vi "gyro -- async fitter.vi"(11 "server event pair":T9) -> ()   [LabVIEW 2018]
uses:
  plot refs -- filter related.ctl
  cursor window action.ctl
  publisher action.ctl
  cursor action.ctl
  2Dwindow.ctl
  server talkback message type.ctl
  circle corners.ctl
  lorentzian.ctl
  peak -- parameters -- complex fit.ctl
  wavepacket.ctl
  filter method control.ctl
  show-win- control.ctl
  server talkto message type.ctl
  server talk-to-back pair.ctl
panel:
  in  "Tab :  Fit controls":T1(tab)
  out "lorentzian":T2={"A (VHz)"=0.005614170164837037, "f (Hz)"=70488.63611178169, "G (Hz)"=428.0110281609372, "phi(rad)"=4.459926465221261, "Q"=164.68883153467982, "Norm  Ampl"=nan, "bg (V)"=2.8688017502385223e-05+0.00035144607353619194i, "4corners"={"z (-pi/2)"=1.2710482317097233e-05+0.00034202144845651717i, "z(inf)"=2.8688017502385223e-05+0.00035144607353619194i, "z (pi/2)"=1.9263392422710455e-05+0.00036742360872147993i, "z center"=1.5986937369903844e-05+0.00035472252858899855i, "z(0)"=3.2858572374224653e-06+0.00035799898364180516i, "radius"=1.3116882032128489e-05}} {"bg (V)" format="%#9_9f"; "Q" format="%#9_9f"; "phi(rad)" format="%#9_9f"; "G (Hz)" format="%#9_9f"; "f (Hz)" format="%#9_9f"}
  in  "Plot: fragment - filter":cluster{dbl[], dbl[]}[](graph)=[{array[298 elements], array[298 elements]}, {array[298 elements], array[298 elements]}, {array[298 elements], array[298 elements]}, {array[298 elements], array[298 elements]}]
  out "Plot: phase around center":cluster{dbl[], dbl[]}[](graph)
  out "Plot: fragment":cluster{dbl[], dbl[]}[](graph)
  out "Plot: complex plane":cluster{dbl[], dbl[]}[](graph)=[{array[298 elements], array[298 elements]}, {[2.9103819402032333e-05, 2.900038886938624e-05, 2.8691728432734196e-05, 2.8182705851547014e-05, 2.748134871600537e-05, 2.6598717847107188e-05, 2.5548732860913123e-05, 2.4347952647886086e-05, 2.301531422929684e-05, 2.1571834109086143e-05, 2.0040276831042943e-05, 1.844479596834995e-05, 1.6810553207305906e-05, 1.516332153250178e-05, 1.3529078771457734e-05, 1.1933597908764745e-05, 1.0402040630721545e-05, 8.958560510510845e-06, 7.625922091921602e-06, 6.4251418788945635e-06, 5.375156892700502e-06, 4.492526023802321e-06, 3.791168888260671e-06, 3.28214630707349e-06, 2.9734858704214465e-06, 2.8700553377753553e-06, 2.973485870421448e-06, 3.28214630707349e-06, 3.7911688882606744e-06, 4.492526023802321e-06, 5.3751568927005036e-06, 6.425141878894565e-06, 7.625922091921604e-06, 8.958560510510852e-06, 1.0402040630721552e-05, 1.1933597908764745e-05, 1.3529078771457736e-05, 1.5163321532501782e-05, 1.6810553207305913e-05, 1.844479596834996e-05, 2.004027683104294e-05, 2.1571834109086143e-05, 2.301531422929684e-05, 2.434795264788609e-05, 2.554873286091313e-05, 2.659871784710719e-05, 2.748134871600537e-05, 2.8182705851547017e-05, 2.86917284327342e-05, 2.9000388869386243e-05], [0.00035472252858899855, 0.00035636650982836675, 0.0003579845645015233, 0.00035955117491969353, 0.0003610416347007352, 0.0003624324384035438, 0.0003637016522229001, 0.00036482925989868135, 0.00036579747838424027, 0.00036659103829567386, 0.00036719742471912916, 0.00036760707457847056, 0.0003678135274507033, 0.0003678135274507033, 0.00036760707457847056, 0.00036719742471912916, 0.00036659103829567386, 0.00036579747838424027, 0.00036482925989868135, 0.0003637016522229001, 0.0003624324384035438, 0.0003610416347007352, 0.00035955117491969353, 0.0003579845645015233, 0.00035636650982836675, 0.00035472252858899855, 0.00035307854734963035, 0.0003514604926764738, 0.00034989388225830357, 0.0003484034224772619, 0.0003470126187744533, 0.000345743404955097, 0.00034461579727931575, 0.00034364757879375683, 0.00034285401888232324, 0.00034224763245886794, 0.00034183798259952654, 0.0003416315297272938, 0.0003416315297272938, 0.00034183798259952654, 0.00034224763245886794, 0.00034285401888232324, 0.00034364757879375683, 0.00034461579727931575, 0.000345743404955097, 0.0003470126187744533, 0.0003484034224772619, 0.00034989388225830357, 0.0003514604926764738, 0.00035307854734963035]}, {[2.8688017502385223e-05, 2.7417909489137084e-05, 2.6147801475888948e-05, 2.487769346264081e-05, 2.3607585449392673e-05, 2.2337477436144533e-05, 2.1067369422896394e-05, 1.9797261409648255e-05, 1.852715339640012e-05, 1.7257045383151983e-05, 1.5986937369903844e-05, 1.4716829356655705e-05, 1.3446721343407567e-05, 1.217661333015943e-05, 1.090650531691129e-05, 9.636397303663155e-06, 8.366289290415015e-06, 7.096181277166876e-06, 5.82607326391874e-06, 4.555965250670601e-06], [0.00035144607353619194, 0.0003517737190414726, 0.00035210136454675325, 0.00035242901005203394, 0.00035275665555731456, 0.00035308430106259525, 0.00035341194656787593, 0.00035373959207315656, 0.00035406723757843724, 0.00035439488308371787, 0.00035472252858899855, 0.00035505017409427923, 0.00035537781959955986, 0.00035570546510484054, 0.00035603311061012117, 0.00035636075611540185, 0.00035668840162068254, 0.00035701604712596316, 0.00035734369263124385, 0.0003576713381365245]}, {[1.2710482317097233e-05, 1.3038127822377894e-05, 1.3365773327658556e-05, 1.3693418832939216e-05, 1.4021064338219878e-05, 1.4348709843500539e-05, 1.4676355348781199e-05, 1.5004000854061861e-05, 1.5331646359342523e-05, 1.5659291864623182e-05, 1.5986937369903844e-05, 1.6314582875184506e-05, 1.6642228380465168e-05, 1.6969873885745827e-05, 1.729751939102649e-05, 1.7625164896307148e-05, 1.795281040158781e-05, 1.8280455906868472e-05, 1.8608101412149134e-05, 1.8935746917429793e-05], [0.00034202144845651717, 0.0003432915564697653, 0.00034456166448301344, 0.00034583177249626157, 0.0003471018805095097, 0.0003483719885227579, 0.000349642096536006, 0.00035091220454925415, 0.0003521823125625023, 0.0003534524205757504, 0.00035472252858899855, 0.0003559926366022467, 0.0003572627446154948, 0.00035853285262874295, 0.0003598029606419911, 0.0003610730686552392, 0.0003623431766684874, 0.00036361328468173553, 0.00036488339269498366, 0.0003661535007082318]}, {[-0.12051735461029346, -0.12207348598889368, -0.12355331127335088, -0.1249559056210327, -0.1262803924561282, -0.1275259440174794, -0.12869178187590485, -0.12977717742069275, -0.13078145231495877, -0.1317039789195845, -0.1325441806854716, -0.13330153251386614, -0.13397556108452827, -0.13456584515154188, -0.13507201580657965, -0.13549375670945876, -0.13583080428584318, -0.13608294789196904, -0.13625002994629012, -0.13633194602796123], [0.06411190542991022, 0.061078796354348035, 0.05800773584383981, 0.05490064321123721, 0.0517594602882955, 0.04858615021209154, 0.045382696198127265, 0.04215110030088447, 0.03889338216260588, 0.03561157775108473, 0.03230773808725083, 0.02898392796334944, 0.02564222465251332, 0.022284716610534536, 0.018913502170647845, 0.015530688232140346, 0.012138388943608257, 0.008738724381682807, 0.005333819226051277, 0.0019258014316016106]}, {[-0.13377675222220706, -0.1355040580524533, -0.1371466641182008, -0.1387035438441276, -0.14017372423108362, -0.14155628646418342, -0.1428503664870357, -0.14405515554175027, -0.14516990067438554, -0.14619390520552009, -0.14712652916565477, -0.14796718969517272, -0.14871536140860767, -0.14937057672299278, -0.1499324261500847, -0.15040055855228054, -0.15077468136206723, -0.15105456076486692, -0.15124002184516333, -0.15133094869581826], [0.07112534787775143, 0.0677585968038774, 0.06434971963721327, 0.06090084681502438, 0.05741413377055908, 0.05389175958597269, 0.050335925630472345, 0.04674885418453284, 0.0431327870510436, 0.03948998415425513, 0.0358227221273995, 0.032133292889868964, 0.02842400221484086, 0.024697168288244413, 0.020955120259970185, 0.01720019678822686, 0.013434744577956244, 0.009661116914218993, 0.005881672191467993, 0.0020987724396288633]}, {array[298 elements], array[298 elements]}]
  in  "scale gauge: Plot: complex plane":dbl(slide)=0.00275 min=0.0 max=0.3 step=1e-06 scale=1e-05..0.5 scale format="%#_3p"
  out "Plot: phase":cluster{"omega out":dbl[], dbl[]}(graph)
  out "Plot: win omega":T4(graph)
  out "Plot: dz/domega":cluster{"omega out":dbl[], dbl[]}(graph)
  in  "Plot: complex plane - filter":cluster{dbl[], dbl[]}[](graph)=[{array[298 elements], array[298 elements]}, {array[298 elements], array[298 elements]}, {[2.905030396515612e-05, 2.9022632451479088e-05, 2.893972711727057e-05, 2.8801915152008838e-05, 2.8609740436560477e-05, 2.8363961396731098e-05, 2.8065548010105136e-05, 2.77156779779875e-05, 2.731573207755454e-05, 2.6867288712557366e-05, 2.6372117684083335e-05, 2.5832173205959713e-05, 2.5249586192364487e-05, 2.4626655848081624e-05, 2.3965840594590203e-05, 2.326974836779799e-05, 2.2541126325709838e-05, 2.1782850006650124e-05, 2.099791198082668e-05, 2.018941004002336e-05, 1.9360534972031112e-05, 1.8514557968066298e-05, 1.7654817712873437e-05, 1.6784707208461826e-05, 1.5907660383476688e-05, 1.5027138541051666e-05, 1.4146616698626644e-05, 1.3269569873641507e-05, 1.2399459369229891e-05, 1.1539719114037038e-05, 1.0693742110072223e-05, 9.864867042079974e-06, 9.056365101276651e-06, 8.271427075453208e-06, 7.513150756393494e-06, 6.784528714305347e-06, 6.088436487513131e-06, 5.427621234021711e-06, 4.804690889738847e-06, 4.222103876143618e-06, 3.682159398019999e-06, 3.1869883695459693e-06, 2.7385450045487964e-06, 2.338599104115837e-06, 1.988729071998198e-06, 1.690315685372236e-06, 1.4445366455428568e-06, 1.252361930094499e-06, 1.1145499648327652e-06, 1.0316446306242462e-06, 1.0039731169472153e-06, 1.0316446306242462e-06, 1.1145499648327669e-06, 1.252361930094499e-06, 1.4445366455428568e-06, 1.6903156853722394e-06, 1.9887290719982014e-06, 2.338599104115837e-06, 2.738545004548798e-06, 3.186988369545971e-06, 3.6821593980200005e-06, 4.2221038761436245e-06, 4.8046908897388484e-06, 5.427621234021715e-06, 6.088436487513134e-06, 6.784528714305345e-06, 7.513150756393502e-06, 8.27142707545321e-06, 9.05636510127666e-06, 9.864867042079978e-06, 1.0693742110072223e-05, 1.1539719114037043e-05, 1.2399459369229895e-05, 1.3269569873641516e-05, 1.4146616698626647e-05, 1.5027138541051664e-05, 1.5907660383476695e-05, 1.6784707208461826e-05, 1.7654817712873447e-05, 1.8514557968066298e-05, 1.936053497203111e-05, 2.0189410040023365e-05, 2.099791198082668e-05, 2.178285000665013e-05, 2.254112632570984e-05, 2.3269748367798e-05, 2.396584059459021e-05, 2.4626655848081624e-05, 2.5249586192364494e-05, 2.5832173205959716e-05, 2.6372117684083342e-05, 2.6867288712557366e-05, 2.731573207755454e-05, 2.77156779779875e-05, 2.806554801010514e-05, 2.83639613967311e-05, 2.860974043656048e-05, 2.8801915152008838e-05, 2.893972711727057e-05, 2.9022632451479088e-05], [0.0003546065647290071, 0.00035548708657143213, 0.00035636413339641725, 0.00035723424390082884, 0.00035809398415602173, 0.0003589399611599865, 0.0003597688362279788, 0.0003605773381687821, 0.00036136227619460554, 0.00036212055251366525, 0.0003628491745557534, 0.0003635452667825456, 0.00036420608203603704, 0.0003648290123803199, 0.00036541159939391515, 0.00036595154387203876, 0.0003664467149005128, 0.00036689515826550997, 0.0003672951041659429, 0.0003676449741980606, 0.00036794338758468654, 0.0003681891666245159, 0.00036838134133996425, 0.000368519153305226, 0.0003686020586394345, 0.00036862973015311157, 0.0003686020586394345, 0.000368519153305226, 0.00036838134133996425, 0.0003681891666245159, 0.00036794338758468654, 0.0003676449741980606, 0.0003672951041659429, 0.00036689515826550997, 0.0003664467149005128, 0.00036595154387203876, 0.00036541159939391515, 0.0003648290123803199, 0.00036420608203603704, 0.0003635452667825456, 0.0003628491745557534, 0.00036212055251366525, 0.00036136227619460554, 0.0003605773381687821, 0.0003597688362279788, 0.0003589399611599865, 0.00035809398415602173, 0.00035723424390082884, 0.00035636413339641725, 0.00035548708657143213, 0.0003546065647290071, 0.00035372604288658204, 0.0003528489960615969, 0.00035197888555718533, 0.00035111914530199244, 0.00035027316829802765, 0.0003494442932300354, 0.0003486357912892321, 0.00034785085326340863, 0.0003470925769443489, 0.00034636395490226076, 0.00034566786267546857, 0.00034500704742197714, 0.00034438411707769426, 0.00034380153006409903, 0.0003432615855859754, 0.0003427664145575014, 0.0003423179711925042, 0.00034191802529207125, 0.0003415681552599536, 0.00034126974187332764, 0.0003410239628334983, 0.0003408317881180499, 0.0003406939761527882, 0.0003406110708185797, 0.0003405833993049026, 0.0003406110708185797, 0.0003406939761527882, 0.0003408317881180499, 0.0003410239628334983, 0.00034126974187332764, 0.0003415681552599536, 0.00034191802529207125, 0.0003423179711925042, 0.0003427664145575014, 0.0003432615855859754, 0.00034380153006409903, 0.00034438411707769426, 0.00034500704742197714, 0.00034566786267546857, 0.00034636395490226076, 0.0003470925769443489, 0.00034785085326340863, 0.0003486357912892321, 0.0003494442932300354, 0.00035027316829802765, 0.00035111914530199244, 0.00035197888555718533, 0.0003528489960615969, 0.00035372604288658204]}, {[3.4550485346656053e-06, -7.59654128881755e-06, 4.382620039101754e-06], [-5.3982458510331535e-06, 1.2688424660565133e-06, -1.3270376410500222e-06]}, {[3.6013253466750408e-06, 3.652728139630199e-06, 3.704130932585357e-06, 3.7555337255405156e-06, 3.806936518495674e-06, 3.858339311450832e-06, 3.909742104405991e-06, 3.961144897361148e-06, 4.012547690316307e-06, 4.063950483271465e-06, 4.115353276226624e-06, 4.166756069181782e-06, 4.21815886213694e-06, 4.269561655092099e-06, 4.320964448047256e-06, 4.372367241002415e-06, 4.423770033957573e-06, 4.475172826912732e-06, 4.52657561986789e-06, 4.5779784128230484e-06], [-4.818979876248634e-06, -4.62743245445747e-06, -4.435885032666307e-06, -4.244337610875143e-06, -4.0527901890839785e-06, -3.861242767292814e-06, -3.669695345501651e-06, -3.478147923710487e-06, -3.2866005019193234e-06, -3.0950530801281598e-06, -2.9035056583369957e-06, -2.711958236545832e-06, -2.5204108147546683e-06, -2.3288633929635042e-06, -2.1373159711723406e-06, -1.9457685493811765e-06, -1.7542211275900128e-06, -1.5626737057988492e-06, -1.371126284007685e-06, -1.1795788622165214e-06]}, {[-7.59654128881755e-06, -7.4016964168323305e-06, -7.206851544847112e-06, -7.012006672861892e-06, -6.817161800876673e-06, -6.6223169288914536e-06, -6.427472056906234e-06, -6.232627184921015e-06, -6.0377823129357955e-06, -5.842937440950577e-06, -5.648092568965357e-06, -5.453247696980138e-06, -5.2584028249949185e-06, -5.063557953009699e-06, -4.86871308102448e-06, -4.6738682090392604e-06, -4.479023337054041e-06, -4.284178465068822e-06, -4.089333593083603e-06, -3.894488721098383e-06], [1.2688424660565133e-06, 1.2688424660565133e-06, 1.2688424660565133e-06, 1.2688424660565133e-06, 1.2688424660565133e-06, 1.2688424660565133e-06, 1.2688424660565133e-06, 1.2688424660565133e-06, 1.2688424660565133e-06, 1.2688424660565133e-06, 1.2688424660565133e-06, 1.2688424660565133e-06, 1.2688424660565133e-06, 1.2688424660565133e-06, 1.2688424660565133e-06, 1.2688424660565133e-06, 1.2688424660565133e-06, 1.2688424660565133e-06, 1.2688424660565133e-06, 1.2688424660565133e-06]}]
  in  "parameters -- scan monitor control.ctlparameters: complex fit":T5={"main VI path"=path "", "scale factor"=3.0, "# of grid points"=200, "parameters: wavepacket"={"R"=0.5, "wave number"=22.0, "delta k"=7.0, "radii vector"=[], "radial section"=[], "wave vector"=22.0, "wavepacket is"=TRUE}, "span"=0.27789, "interference ?"=enum."cp z center", "filter method"=enum."three"} {"span" min=0.0 max=0.5 step=1e-05 scale=0.0001..0.5 scale format="%#_5f"; "parameters: wavepacket"."delta k" format="%#_3f"; "parameters: wavepacket"."wave number" format="%#_3f"; "parameters: wavepacket"."R" format="%#_3f"}
  in  "win":T8={"cen (Hz)"=45005.0594236074, "win (Hz)"=127.23590686512762, "left (Hz)"=44941.44147017484, "right (Hz)"=45068.67737703997}
  out "circle frequency (Hz)":dbl=70488.63611178169 format="%#11_11f"
  out "circle gamma (Hz)":dbl=428.0110281609372 format="%#11_11f"
  out "circle phase (rad)":dbl=4.459926465221261 format="%#11_11f"
  out "circle Q":dbl=164.68883153467982 format="%#11_11f"
  in  "tab":enum32{"complex plane"}(tab)
  in  "plot staff!":enum16{"plot", "do not plot", "a"}(ring)
  in  "use fast fit!":bool
  out "# of points":dbl=953.475933538175
  out "win center (kHz)":dbl=3399.029286744401
  out "win width (kHz)":dbl=76.27809365793496
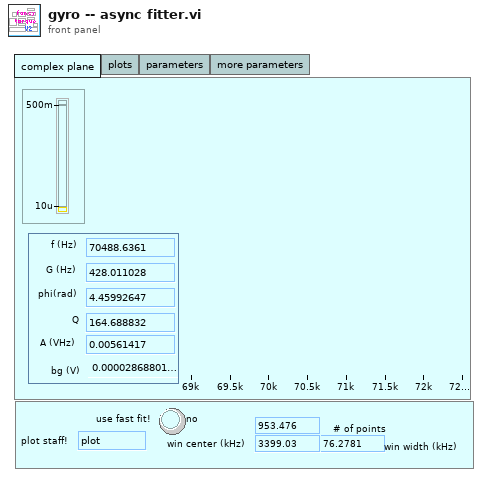
[diagram p1: front panel]
types:
  T1 = enum32{"complex plane", "plots", "parameters", "more parameters"}
  T2 = typedef "lorentzian.ctl" = cluster{"A (VHz)":dbl, "f (Hz)":dbl, "G (Hz)":dbl, "phi(rad)":dbl, "Q":dbl, "Norm  Ampl":dbl, "bg (V)":cdb, "4corners":T3}
  T3 = typedef "circle corners.ctl" = cluster{"z (-pi/2)":cdb, "z(inf)":cdb, "z (pi/2)":cdb, "z center":cdb, "z(0)":cdb, "radius":dbl}
  T4 = cluster{"omega out":dbl[], "win omega out":dbl[]}
  T5 = typedef "peak -- parameters -- complex fit.ctl" = cluster{"main VI path":path, "scale factor":dbl, "# of grid points":i32, "parameters: wavepacket":T6, "span":dbl, "interference ?":enum16{"cp z center", "pm zcenter", "fancy"}, "filter method":T7}
  T6 = typedef "wavepacket.ctl" = cluster{"R":dbl, "wave number":dbl, "delta k":dbl, "radii vector":dbl[], "radial section":cdb[], "wave vector":dbl, "wavepacket is":bool}
  T7 = typedef "filter method control.ctl" = enum16{"four", "five", "one", "two", "three", "zero", "minus one", "minus two"}
  T8 = typedef "show-win- control.ctl" = cluster{"cen (Hz)":dbl, "win (Hz)":dbl, "left (Hz)":dbl, "right (Hz)":dbl}
  T9 = typedef "server talk-to-back pair.ctl" = cluster{"talkback event":refnum<user-event>, "talkto event":refnum<user-event>}
  T10 = typedef "plot refs -- filter related.ctl" = cluster{"Plot: complex plane - filter":refnum<vi>, "Plot: dz/domega":refnum<vi>, "Plot: fragment filter":refnum<vi>, "Plot: win omega":refnum<vi>, "Plot: phase":refnum<vi>, "Plot: phase around center":refnum<vi>, "Plot: complex plane":refnum<vi>, "Plot: fragment":refnum<vi>}
  T11 = typedef "2Dwindow.ctl" = cluster{"window y":dbl, "center x":dbl, "center y":dbl, "window x":dbl}
  T12 = typedef "cursor action.ctl" = enum16{"range", "read", "write", "check", "zoom out", "smart zoom out", "zoom to aspect ratio 1", "zoom to win", "zoom out 20%", "zoom in 20%", "-empty", "smart zoom out&aspect", "move range left 20%", "move range right 20%", "move range up 20%", "move range down 20%", "zoom to X win", "zoom to Y win", "zoom out X", "zoom out Y", "zoom in X", "zoom in Y", "check plot scale"}
  T13 = typedef "cursor window action.ctl" = enum16{"balance", "h. offset change", "cursor moves", "change center", "change window", "init", "check", "reset", "set y to middle", "idle", "-write all Y", "-write left.X", "-write center.X", "-write right.X", "-write all X", "-change center", "-change window", "-change skew", "-read cursor 2", "-read cursor 1", "-read cursor 0", "-read all cursors", "-reset", "-read plot scale", "-set y to middle", "-Q: center.Y is visible", "-Q: window is visible", "-parse center.Y", "-right left from center", "-left move", "-right move", "-set center.Y", "-empty", "-set cursors to default", "-check", "-write center.Y", "-copy cursor 1", "-copy cursor 0", "-copy cursor 2", "move right", "move left", "shrink", "broaden", "skew up", "skew down", "-write plot scale", "zoom X", "change cen&win", "zoom to all data", "color--red", "color--green", "color--yellow", "read", "zoom out", "zoom in", "slide right", "slide left", "set range aspect ratio to 1"}
  T14 = typedef "eventvkey.ctl" = enum16{"ASCII", "Enter", "Return", "Shift", "Ctrl", "Alt", "Cmd", "Opt", "Caps", "NumLock", "Clear", "Break", "Up", "Down", "Left", "Right", "Insert", "Delete", "Home", "End", "PageUp", "PageDown", "Escape", "Help", "Pause", "ScrollLock", "F1", "F2", "F3", "F4", "F5", "F6", "F7", "F8", "F9", "F10", "F11", "F12", "F13", "F14", "F15", "F16", "F17", "F18", "F19", "F20", "F21", "F22", "F23", "F24", "Play", "VolumeUp", "VolumeDown", "Mute", "Two Byte Char"}
  T15 = typedef "publisher action.ctl" = enum16{"set", "get", "init", "check"}
  T16 = typedef "server talkback message type.ctl" = cluster{"message":enum16{"new", "void"}}
  T17 = typedef "cursor winow.ctl" = cluster{"left":dbl, "right ":dbl, "center":dbl, "window":dbl, "cursors":i32[], "relative":i32, "absolute":i32, "fixed vertical offset":dbl, "vertical offset":dbl, "skew":dbl, "default window frac":dbl, "kind":enum16{"symmetric", "skewed", "fancy"}, "skew.left":dbl, "skew.right":dbl, "Plot ref":refnum<vi>, "wing order":enum16{"forw", "back"}}
  T18 = enum16{"stop", "start", "update pars", "update request", "new", "launch", "exit", "get", "reset", "pause", "unpause"}
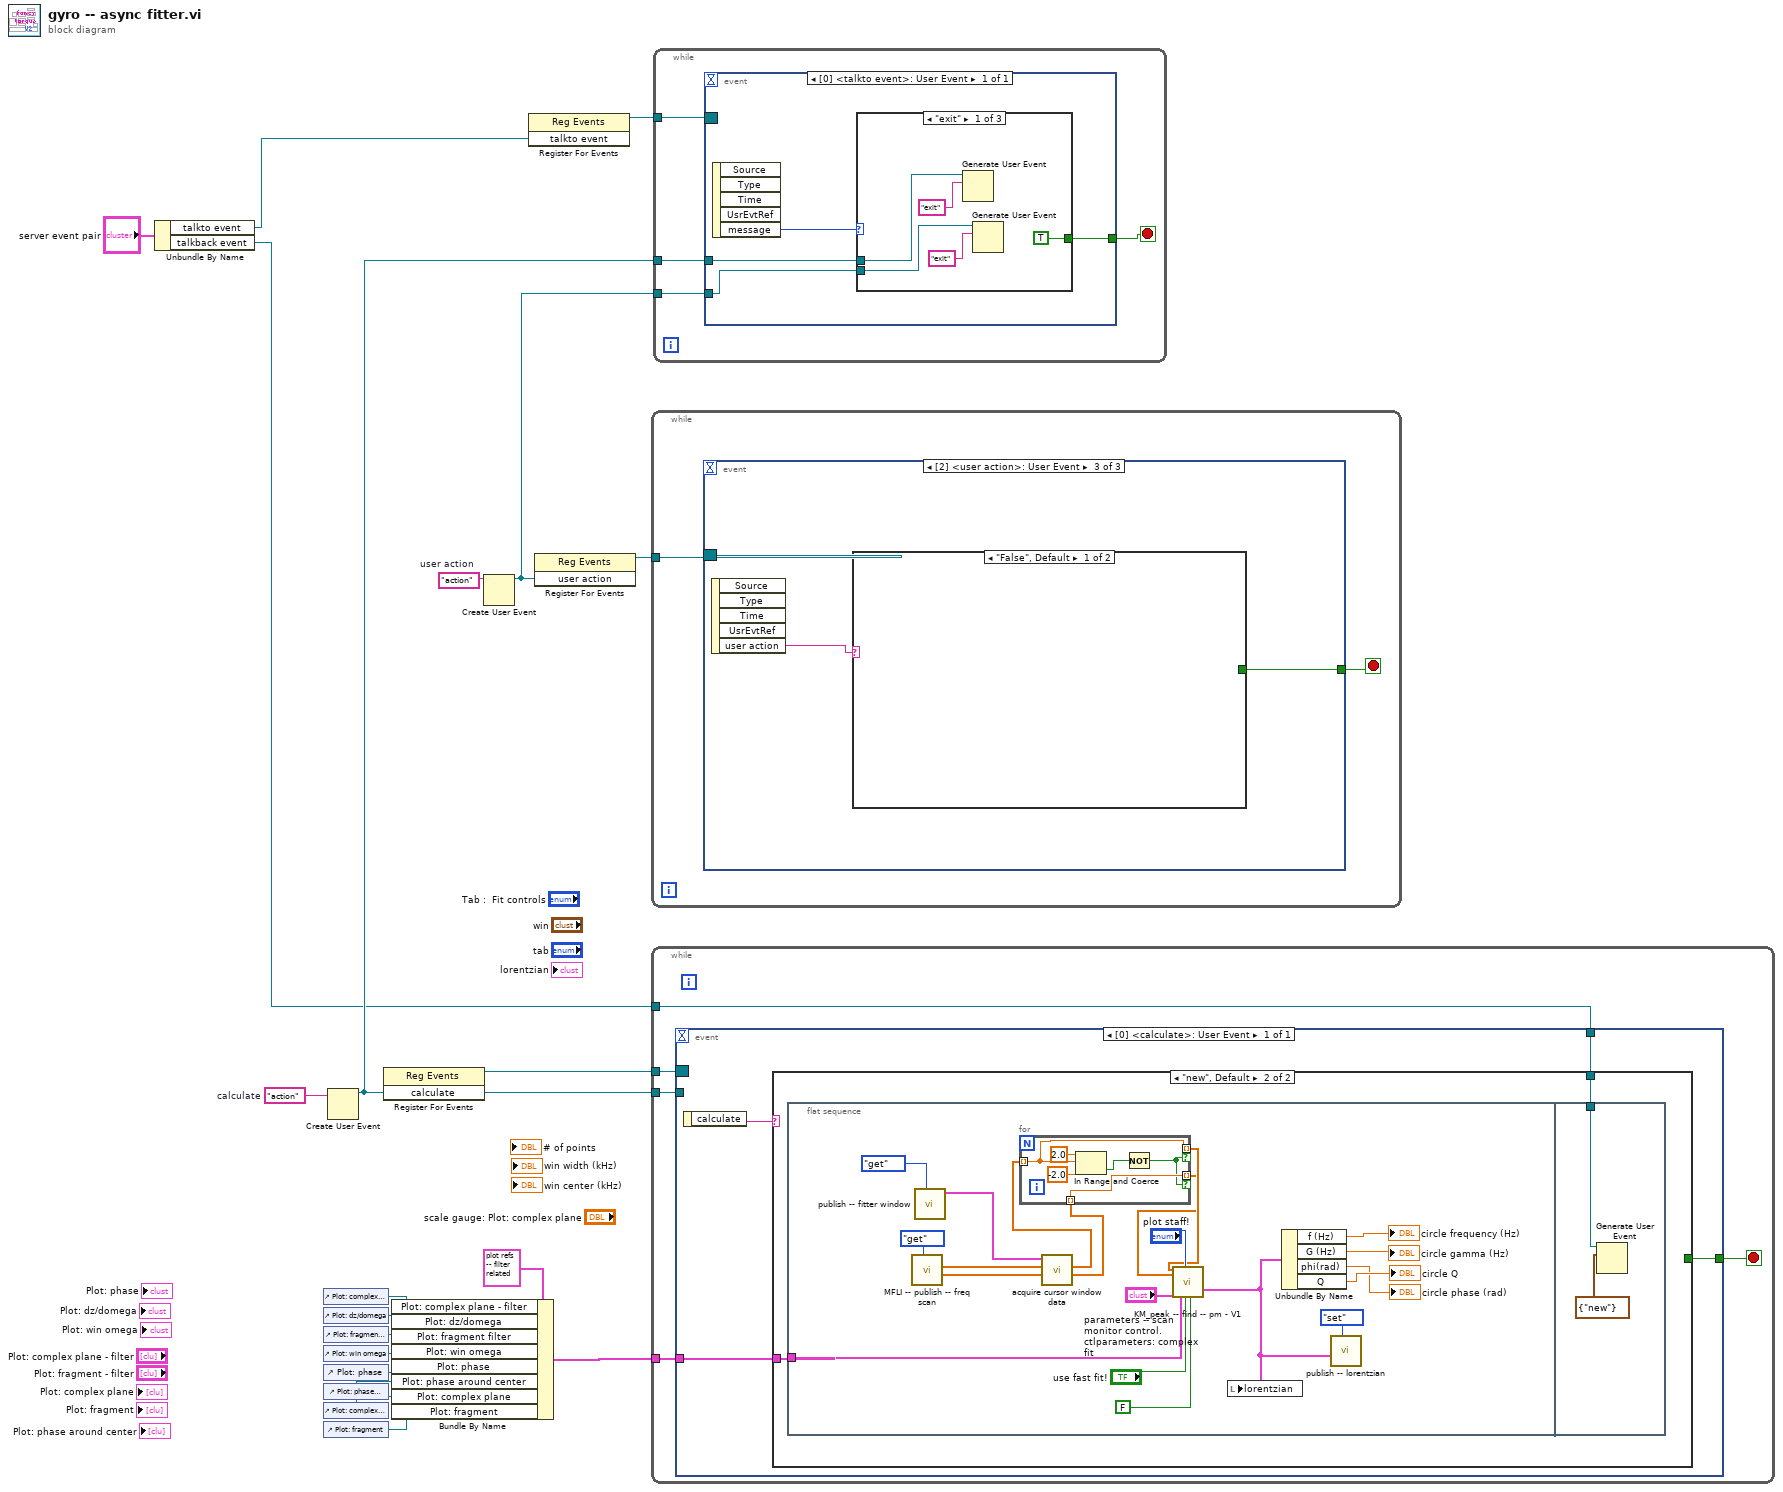
[diagram p0: block diagram]
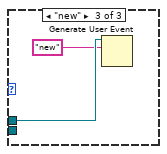
[diagram p3: hidden frame]
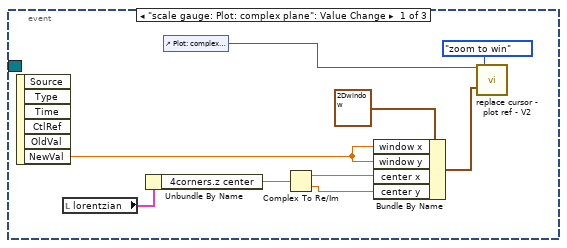
[diagram p4: hidden frame]
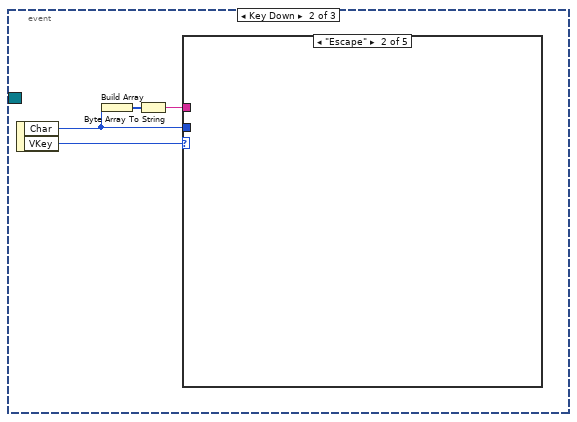
[diagram p5: hidden frame]
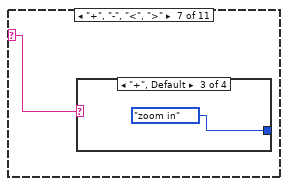
[diagram p13: hidden frame]
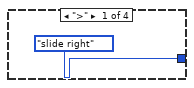
[diagram p14: hidden frame]
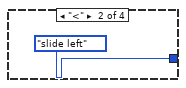
[diagram p15: hidden frame]
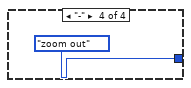
[diagram p16: hidden frame]
diagram:
  w17 = "action"  # user action
  w19 = "action"  # calculate
  n1 = Unbundle By Name("server event pair") -> ("talkto event"=w3:refnum<user-event>, "talkback event"=w2:refnum<user-event>)
  n2 = control-ref of="Plot: complex plane - filter"() -> (w15:refnum<vi>)
  n3 = control-ref of="Plot: dz/domega"() -> (w14:refnum<vi>)
  n4 = control-ref of="Plot: fragment - filter"() -> (w13:refnum<vi>)
  n5 = control-ref of="Plot: win omega"() -> (w12:refnum<vi>)
  n6 = control-ref of="Plot: phase"() -> (w11:refnum<vi>)
  n7 = control-ref of="Plot: phase around center"() -> (w9:refnum<vi>)
  n8 = control-ref of="Plot: complex plane"() -> (w8:refnum<vi>)
  n9 = control-ref of="Plot: fragment"() -> (w7:refnum<vi>)
  n10 = Create User Event(user event datatype=w19) -> (user event=w5:refnum<user-event>)  [unwired: 1 in, 1 out]
  n11 = register-events(w5) -> (reference out=w20:refnum<event-registration>)  [unwired: 2 in, 1 out]
  n12 = Bundle By Name(cluster=T10 {"Plot: complex plane - filter"=refnum, "Plot: dz/domega"=refnum, "Plot: fragment filter"=refnum, "Plot: win omega"=refnum, "Plot: phase"=refnum, "Plot: phase around center"=refnum, "Plot: complex plane"=refnum, "Plot: fragment"=refnum} ("plots: filter related"), "Plot: complex plane - filter"=w15, "Plot: dz/domega"=w14, "Plot: fragment filter"=w13, "Plot: win omega"=w12, "Plot: phase"=w11, "Plot: phase around center"=w9, "Plot: complex plane"=w8, "Plot: fragment"=w7) -> (w10:T10)
  n13 = Create User Event(user event datatype=w17) -> (user event=w1:refnum<user-event>)  [unwired: 1 in, 1 out]
  n14 = register-events(w3) -> (reference out=w6:refnum<event-registration>)  [unwired: 2 in, 1 out]
  n15 = register-events(w1) -> (reference out=w18:refnum<event-registration>)  [unwired: 2 in, 1 out]
  n16 = while {
    tunnel: w18 -> [w22]
    stop <- w21 stop-if-true
    n17 = event shown="[2] <user action>: User Event" {
      selector: w22 -> [_ _ _]
      dyn-events: _ -> [_ _ _]
      timeout: _ -> [_ _ _]
      tunnel: [_ _ w47] -> w21
      event "scale gauge: Plot: complex plane": Value Change {
        n18 = event-data() -> ("NewVal"=w25:dbl)  [unwired: 1 in, 5 out]
        n19 = local read "lorentzian"() -> (w23:T2)
        n20 = Unbundle By Name(w23) -> ("4corners.z center"=w31:cdb)
        n21 = control-ref of="Plot: complex plane"() -> (w30:refnum<vi>)
        n22 = Complex To Re/Im(x + iy=w31) -> (x=w27:dbl, y=w26:dbl)
        n23 = Bundle By Name(cluster=T11 {"window y"=0.0021014740628288917, "center x"=44850.89441339177, "center y"=2.5658109925320947, "window x"=17480.201988350764} ("window IN"), "window x"=w25, "window y"=w25, "center x"=w27, "center y"=w26) -> (w24:T11)
        n24 = call "replace cursor - plot ref - V2.vi"("Plot ref in"=w30, "window IN"=w24, "cursor action"=cursor_action."zoom to win") -> ()  [unwired: 13 in, 4 out]
      }
      event Key Down {
        n25 = event-data() -> ("Char"=w33:i16, "VKey"=w35:T14)  [unwired: 1 in]
        n26 = Build Array(w33) -> (w34:i16[])
        n27 = Byte Array To String(unsigned byte array=w34) -> (string=w32:string)
        n28 = case shown="\"Escape\"" w35 {
          selector: w35 -> [_ _ _ _ w42]
          tunnel: w33 -> [_ _ _ _ _]
          tunnel: w32 -> [w36 _ _ _ _]
          frame "ASCII", Default {
            n29 = case shown="\"d\"" w36 {
              selector: w36 -> [_ _ _ _ _ _ w37 _ _ _ _]
              frame "0", Default {
              }
              frame "a" {
              }
              frame "s" {
              }
              frame "l" {
              }
              frame "p" {
              }
              frame "?" {
              }
              frame "+", "-", "<", ">" {
                n30 = case shown="\"+\", Default" w37 {
                  tunnel: [cursor_window_action."slide right" ("cursor window action") cursor_window_action."slide left" ("cursor window action") cursor_window_action."zoom in" ("cursor window action") cursor_window_action."zoom out" ("cursor window action")] -> _
                  frame ">" {
                  }
                  frame "<" {
                  }
                  frame "+", Default {
                  }
                  frame "-" {
                  }
                }
              }
              frame "c" {
              }
              frame "t" {
              }
              frame "r" {
              }
              frame "d" {
              }
            }
          }
          frame "Escape" {
          }
          frame "PageUp" {
          }
          frame "PageDown" {
          }
          frame "Up".."Right" {
            n31 = case shown="\"Left\"" w42 {
              tunnel: [cursor_window_action."move right" ("cursor window action") cursor_window_action."move left" ("cursor window action") cursor_window_action."broaden" ("cursor window action") cursor_window_action."shrink" ("cursor window action")] -> _
              frame "Right", Default {
              }
              frame "Left" {
              }
              frame "Up" {
              }
              frame "Down" {
              }
            }
          }
        }
      }
      event User Event {
        n32 = event-data() -> ("user action"=w48:string)  [unwired: 1 in, 4 out]
        n33 = case shown="\"False\", Default" w48 {
          tunnel: [_ TRUE] -> w47
          frame "False", Default {
          }
          frame "exit" {
          }
        }
      }
    }
  }
  n34 = while {
    tunnel: w20 -> [w54]
    tunnel: w5 -> [w53]
    tunnel: w10 -> [w52]
    tunnel: w2 -> [w51]
    stop <- w50 stop-if-true
    n35 = event shown="[0] <calculate>: User Event" {
      selector: w54 -> [_]
      dyn-events: _ -> [_]
      timeout: _ -> [_]
      tunnel: w53 -> [_]
      tunnel: w52 -> [w58]
      tunnel: w51 -> [w57]
      tunnel: [w55] -> w50
      event User Event {
        n36 = event-data() -> ("calculate"=w56:string)  [unwired: 1 in]
        n37 = case shown="\"new\", Default" w56 {
          tunnel: w58 -> [_ w61]
          tunnel: w57 -> [_ w60]
          tunnel: [TRUE _] -> w55
          frame "exit" {
          }
          frame "new", Default {
            n38 = flat-sequence {
              tunnel: w61 -> [w81]
              tunnel: w60 -> [w89]
              frame #0 {
                n39 = call "MFLI -- publish -- freq scan.vi"("publisher action"=publisher_action."get") -> ("Voltage out (V)"=w68:cdb[], "Freq out (Hz)"=w69:dbl[])  [unwired: 9 in]
                n40 = call "publish -- fitter window.vi"("publisher action"=publisher_action."get") -> ("win OUT"=w66:T17)  [unwired: 10 in]
                n41 = call "acquire cursor window data.vi"("z in"=w68, "omega in"=w69, "cursor window"=w66) -> ("z out"=w64:cdb[], "omega  out"=w65:dbl[])  [unwired: 4 in, 3 out]
                n42 = for {
                  tunnel: w65 -> [w84] mode=indexing
                  tunnel: w64 -> [w85] mode=indexing
                  tunnel: [w85] -> w62 mode=indexing if=w82
                  tunnel: [w84] -> w63 mode=indexing if=w82
                  n43 = In Range and Coerce(upper limit=2.0, x=w84, lower limit=-2.0) -> (In Range?=w83:bool)  [unwired: 1 out]
                  n44 = Not(x=w83) -> (.not. x?=w82:bool)
                }
                n45 = call "KM_peak -- find -- pm - V1.vi"("omega in"=w63, "z in"=w62, "parameters: complex fit"="parameters -- scan monitor control.ctlparameters: complex fit", "plots: filter related"=w81, "plot staff ?"="plot staff!", "just guess?"="use fast fit!", "subtract linear BG"=FALSE) -> ("pm lorentzian"=w71:T2)  [unwired: 10 in, 2 out]
                n46 = local write "lorentzian"(w71) -> ()
                n47 = Unbundle By Name(w71) -> ("f (Hz)"=→"circle frequency (Hz)":dbl, "G (Hz)"=→"circle gamma (Hz)":dbl, "phi(rad)"=→"circle phase (rad)":dbl, "Q"=→"circle Q":dbl)
                n48 = call "publish -- lorentzian.vi"("publisher action"=publisher_action."set", "lorentzian IN"=w71) -> ()  [unwired: 9 in, 1 out]
              }
              frame #1 {
                n49 = Generate User Event(user event=w89, event data cluster=T16 {"message"=enum."new"} ("event data")) -> ()  [unwired: 2 in, 2 out]
              }
            }
          }
        }
      }
    }
  }
  n50 = while {
    tunnel: w6 -> [w93]
    tunnel: w5 -> [w91]
    tunnel: w1 -> [w90]
    stop <- w92 stop-if-true
    n51 = event shown="[0] <talkto event>: User Event" {
      selector: w93 -> [_]
      dyn-events: _ -> [_]
      timeout: _ -> [_]
      tunnel: [w96] -> w92
      tunnel: w91 -> [w95]
      tunnel: w90 -> [w94]
      event User Event {
        n52 = event-data() -> ("message"=w97:T18)  [unwired: 1 in, 4 out]
        n53 = case shown="\"exit\"" w97 {
          tunnel: [TRUE _ _] -> w96
          tunnel: w95 -> [w101 _ w104]
          tunnel: w94 -> [w98 _ _]
          frame "exit" {
            n54 = Generate User Event(user event=w101, event data cluster="exit" ("event data")) -> ()  [unwired: 2 in, 2 out]
            n55 = Generate User Event(user event=w98, event data cluster="exit" ("event data")) -> ()  [unwired: 2 in, 2 out]
          }
          frame "start", Default {
          }
          frame "new" {
            n56 = Generate User Event(user event=w104, event data cluster="new" ("event data")) -> ()  [unwired: 2 in, 2 out]
          }
        }
      }
    }
  }
